vi "ble_write_by_handle.vi"   [LabVIEW 2015]
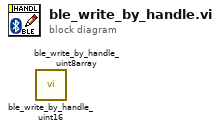
[diagram p0: block diagram]
diagram:
  n1 = call "ble_write_by_handle_uint16.vi"() -> ()  [unwired: 10 in, 2 out]
  n2 = call "ble_write_by_handle_uint8array.vi"() -> ()  [unwired: 10 in, 2 out]
